vi "PH_SHS_Analysis.ProcPeriodic.vi"(0 "i ref in":refnum<vi>, 3 "ms timeout (10000)":i32=10000, 5 "error in (no error)":errorcluster) -> (14 "i ref out":refnum<vi>, 17 "timed out":bool, 19 "error out":errorcluster)   [LabVIEW 2014, in "PH_SHS_Analysis.lvlib"]
doc: "This method serves to periodically do things like reading values from the HW. Methods that should be executed periodically should be called from THIS methode. Add code here."
uses:
  PH_SHS_Analysis.lvlib
  PH_Basics/PH_StatusHandler/PH_StatusHandler.Status.ctl
  PH_SHS_Analysis.Zernike Dataset.ctl
  PH_SHS_Analysis.Zernike Coefficients.ctl
  PH_Basics/PH_Common/PH_Common.lvlib
  CSlibraries-extern/DimLVEvent/LVDimInterface/LVDimInterface.lvlib
  PH_Basics/PH_Img_BaseClass/PH_Img_BaseClass.lvlib
  PH_Basics/PH_StatusHandler/PH_StatusHandler.lvlib
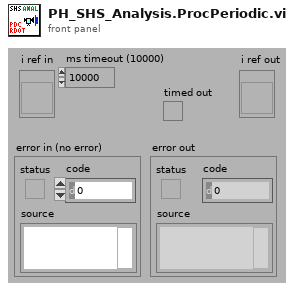
[diagram p1: front panel]
types:
  T1 = typedef "PH_SHS_Analysis.lvlib/PH_SHS_Analysis.Zernike Dataset.ctl" = cluster{"State":T2, "Time Stamp":timestamp, "PtV [lambda]":dbl, "Zernicke Coefficients":T3}
  T2 = typedef "PH_StatusHandler.lvlib/PH_StatusHandler.Status.ctl" = i16
  T3 = typedef "PH_SHS_Analysis.lvlib/PH_SHS_Analysis.Zernike Coefficients.ctl" = cluster{"Tilt x":dbl, "Tilt y":dbl, "Defocus":dbl, "Astig 0°":dbl, "Astig 45°":dbl, "Coma x":dbl, "Coma y":dbl, "Spherical":dbl, "Trefoil 0°":dbl, "Trefoil 30°":dbl, "2nd Astig 0°":dbl, "2nd Astig 45°":dbl, "2nd Coma x":dbl, "2nd Coma y":dbl, "2nd Spherical":dbl}
  T4 = typedef "IMAQ Image.ctl" = refnum<image>
  T5 = typedef "PH_SHS_Analysis.lvlib/PH_SHS_Analysis.i attribute.ctl" = cluster{"GUI Refs":cluster{"Delete":refnum<vi>, "Global On":refnum<vi>, "Cam Source":refnum<vi>, "Calibration Data File":refnum<vi>, "Calibration status":refnum<vi>, "Show overlay":refnum<vi>, "SHS Device Config":refnum<vi>, "Result":refnum<vi>, "Consider Tilt":refnum<vi>, "Working Reference":refnum<vi>, "Remove Tilt":refnum<vi>, "Take Cali  Reference":refnum<vi>, "Publishing Data Status":refnum<vi>, "Calibration Data":refnum<vi>}, "Calibration":cluster{"Status":T2, "Data":T6, "File":path}, "Result":T11, "Image":T4, "SHS Device Config":T13, "Show Overlay":bool, "GradientZernikeMatrix":dbl[][], "Consider Tilt":bool, "Working Reference":T7, "Zernicke Service ID":i32, "PSDB Image":T4}
  T6 = typedef "PH_SHS_Analysis_Calibrator.lvlib/PH_SHS_Analysis_Calibrator.Analysis Calibration Data.ctl" = cluster{"Date":string, "Time":string, "Cam Settings":cluster{"Cam ID":string, "Gain":dbl, "Brightness":dbl, "Shutter":dbl, "Cam Error":bool, "Mode":i32}, "SHS Reference Result":T7, "Pixel Size":dbl, "MLA Pitch":dbl, "Method":enum16{"automatic", "manual"}, "Calibration Data calculated":bool, "No Problems at calculation?":bool, "error out":errorcluster}
  T7 = typedef "SHS_Common.lvlib/SHSReference.ctl" = cluster{"Reference":T8[][], "Lens Array Pitch [px]":dbl}
  T8 = typedef "SHS_Common.lvlib/ReferencePoint.ctl" = cluster{"Rect":T9, "Point":T10}
  T9 = typedef "SHS_Common.lvlib/Rectangle.ctl" = cluster{"Left":i32, "Top":i32, "Right":i32, "Bottom":i32}
  T10 = typedef "SHS_Common.lvlib/Point.ctl" = cluster{"x":dbl, "y":dbl, "valid?":bool, "weight":dbl}
  T11 = typedef "PH_SHS_Analysis.lvlib/PH_SHS_Analysis.Result.ctl" = cluster{"Time Stamp":timestamp, "Zernike Coefficients":T3, "PtV [lambda]":dbl, "Shifts":T12, "Measurement Quality":cluster{dbl, dbl, dbl}, "Measurement valid?":bool}
  T12 = typedef "SHS_Common.lvlib/Shifts.ctl" = T10[][]
  T13 = typedef "SHS_Analysis.lvlib/SHS_DeviceConfig.ctl" = cluster{"focal length [m]":dbl, "pixel size [m/px]":dbl, "wavelength [m]":dbl}
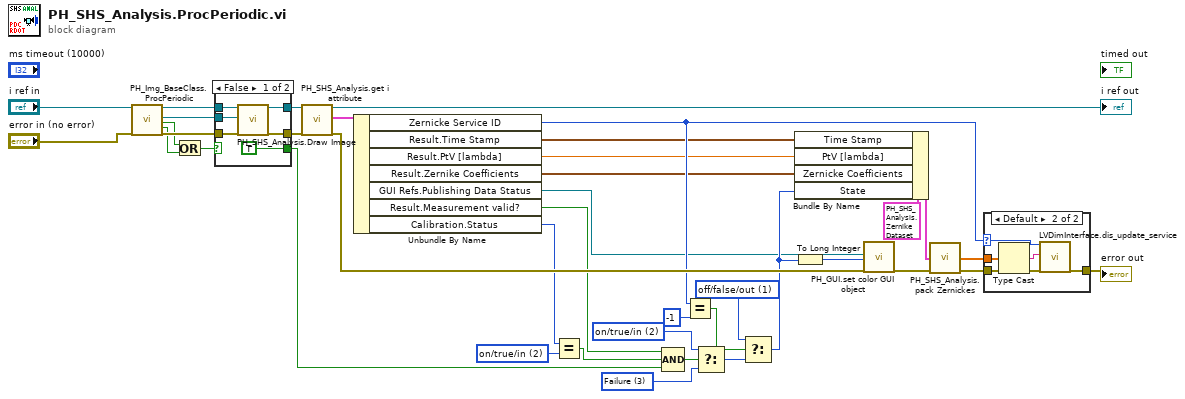
[diagram p0: block diagram]
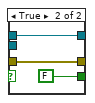
[diagram p3: hidden frame]
diagram:
  w12 = T2 3 items=["no info", "off/false/out", "on/true/in", "Failure", "Alarm", "Status 1", "Status 2", "Status 3"] ("State")
  w13 = T2 2 items=["no info", "off/false/out", "on/true/in", "Failure", "Alarm", "Status 1", "Status 2", "Status 3"] ("State")
  w14 = T2 1 items=["no info", "off/false/out", "on/true/in", "Failure", "Alarm", "Status 1", "Status 2", "Status 3"] ("State")
  w30 = T2 2 items=["no info", "off/false/out", "on/true/in", "Failure", "Alarm", "Status 1", "Status 2", "Status 3"] ("y")
  n1 = call "PH_Img_BaseClass.ProcPeriodic.vi"("i ref in"="i ref in", "error in (no error)"="error in (no error)") -> ("i ref out"=w37:refnum<vi>, "Cam Image"=w2:T4, "timed out?"=w5:bool, "Error while unflatten data?"=w4:bool, "error out"=w7:errorcluster)  [unwired: 13 in]
  n2 = Or(x=w5, y=w4) -> (x .or. y?=w3:bool)
  n3 = case shown="False" w3 {
    tunnel: w37 -> [w43 w46]
    tunnel: [w40 w46] -> w31
    tunnel: w7 -> [w42 w45]
    tunnel: [w41 w45] -> w6
    tunnel: w2 -> [w38 _]
    tunnel: [TRUE FALSE] -> w28
    frame False {
      n4 = call "PH_SHS_Analysis.Draw Image.vi"("i ref in"=w43, "Cam Image"=w38, "error in (no error)"=w42) -> ("i ref out"=w40:refnum<vi>, "error out"=w41:errorcluster)  [unwired: 15 in]
    }
    frame True {
    }
  }
  n5 = call "PH_SHS_Analysis.get i attribute.vi"("i ref in"=w31, "error in (no error)"=w6) -> ("i ref out"=→"i ref out":refnum<vi>, "i attribute"=w19:T5, "error out"=w25:errorcluster)  [unwired: 15 in]
  n6 = Unbundle By Name(w19) -> ("Zernicke Service ID"=w22:i32, "Result.Time Stamp"=w15:timestamp, "Result.PtV [lambda]"=w9:dbl, "Result.Zernike Coefficients"=w8:T3, "GUI Refs.Publishing Data Status"=w10:refnum<vi>, "Result.Measurement valid?"=w20:bool, "Calibration.Status"=w21:T2)
  n7 = Equal?(x=w21, y=w30) -> (x = y?=w29:bool)
  n8 = Compound Arithmetic op=AND(w20, w29, w28) -> (w27:bool)
  n9 = Equal?(x=w22, y=-1) -> (x = y?=w33:bool)
  n10 = Select(t=w13, s=w27, f=w12) -> (s? t:f=w26:T2)
  n11 = Select(t=w14, s=w33, f=w26) -> (s? t:f=w11:T2)
  n12 = Bundle By Name(cluster=T1 {"State"=0, "Time Stamp"=timestamp(0 s since 1904-01-01), "PtV [lambda]"=0.0, "Zernicke Coefficients"={"Tilt x"=0.0, "Tilt y"=0.0, "Defocus"=0.0, "Astig 0°"=0.0, "Astig 45°"=0.0, "Coma x"=0.0, "Coma y"=0.0, "Spherical"=0.0, "Trefoil 0°"=0.0, "Trefoil 30°"=0.0, "2nd Astig 0°"=0.0, "2nd Astig 45°"=0.0, "2nd Coma x"=0.0, "2nd Coma y"=0.0, "2nd Spherical"=0.0}} ("SHS Zernicke Dataset"), "Time Stamp"=w15, "PtV [lambda]"=w9, "Zernicke Coefficients"=w8, "State"=w11) -> (w17:T1)
  n13 = To Long Integer(number=w11) -> (32bit integer=w1:i32)
  n14 = call "PH_GUI.set color GUI object.vi"("GUI object Ref"=w10, "State"=w1, "error in (no error)"=w25) -> ("error out"=w24:errorcluster)  [unwired: 16 in]
  n15 = call "PH_SHS_Analysis.pack Zernickes.vi"("SHS Zernicke Dataset"=w17) -> ("DIM Service Array"=w16:dbl[])
  n16 = case shown="Default" w22 {
    selector: w22 -> [_ w48]
    tunnel: w16 -> [_ w51]
    tunnel: w24 -> [w47 w50]
    tunnel: [w47 w49] -> w23
    frame -1 {
    }
    frame Default {
      n17 = Type Cast(x=w51) -> (*(type *) &x=w52:string)  [unwired: 1 in]
      n18 = call "LVDimInterface.dis_update_service.vi"("my_serviceID"=w48, "data"=w52, "error in (no error)"=w50) -> ("error out"=w49:errorcluster)  [unwired: 14 in, 2 out]
    }
  }
  "error out" <- w23
